vi "GUI_fast.vi"() -> ()   [LabVIEW 2013]
panel:
  out "indecator ref array":refnum<vi>[](array[refnum])
  in  "time to wait (TCP) 2":i32=10
  in  "plot":bool=TRUE
  out "ratio(h)":bool=TRUE
  out "fixsize":bool
  in  "shotnumber":i32
  out "error (h)":bool
  out "Device Name (h)":string="StagingOAP2Far"
  in  "Main Tap":T1(tab)
  in  "centroidx":dbl=453.118958
  in  "centroidy":dbl=178.22908
  out "XY Graph":cluster{u32, "centroidx":dbl}[](graph)=[{52, "centroidx"=458.85675}, {106, "centroidx"=457.702789}, {153, "centroidx"=451.882446}, {204, "centroidx"=452.284454}, {247, "centroidx"=452.532745}, {296, "centroidx"=451.082489}, {346, "centroidx"=459.559479}, {395, "centroidx"=451.41272}, {444, "centroidx"=452.080353}, {489, "centroidx"=451.756592}, {535, "centroidx"=455.360901}, {589, "centroidx"=451.727661}, {632, "centroidx"=457.428375}, {678, "centroidx"=458.708496}, {728, "centroidx"=456.774231}, {784, "centroidx"=457.488647}, {834, "centroidx"=451.875549}, {876, "centroidx"=457.952881}, {926, "centroidx"=459.627014}, {978, "centroidx"=456.600525}, {1024, "centroidx"=450.505829}, {1073, "centroidx"=452.936493}, {1123, "centroidx"=452.39035}, {1170, "centroidx"=452.66568}, {1219, "centroidx"=459.740845}, {1264, "centroidx"=426.268219}, {1316, "centroidx"=457.931732}, {1361, "centroidx"=457.714844}, {1411, "centroidx"=453.192993}, {1460, "centroidx"=456.957214}, {1508, "centroidx"=457.535095}, {1557, "centroidx"=459.828217}, {1602, "centroidx"=458.309296}, {1650, "centroidx"=457.216583}, {1697, "centroidx"=451.62738}, {1748, "centroidx"=457.94928}, {1794, "centroidx"=451.556854}, {1846, "centroidx"=454.358826}, {1890, "centroidx"=452.673492}, {1945, "centroidx"=457.183167}, {1992, "centroidx"=451.190216}, {2040, "centroidx"=457.415009}, {2091, "centroidx"=456.950653}, {2141, "centroidx"=458.052216}, {2186, "centroidx"=459.17218}, {2234, "centroidx"=458.392334}, {2287, "centroidx"=454.510315}, {2326, "centroidx"=458.260986}, {2378, "centroidx"=449.234619}, {2427, "centroidx"=452.183594}, {2473, "centroidx"=457.933685}, {2522, "centroidx"=458.143616}, {2568, "centroidx"=456.90979}, {2625, "centroidx"=453.549866}, {2675, "centroidx"=459.572571}, {2722, "centroidx"=456.521057}, {2768, "centroidx"=457.70401}, {2815, "centroidx"=457.971252}, {2862, "centroidx"=456.893097}, {2911, "centroidx"=452.007233}, {2960, "centroidx"=455.334778}, {3010, "centroidx"=457.899597}, {3057, "centroidx"=460.034424}, {3111, "centroidx"=456.625671}, {3149, "centroidx"=454.197052}, {3200, "centroidx"=453.378296}, {3250, "centroidx"=457.949677}, {3295, "centroidx"=453.204376}, {3349, "centroidx"=458.059357}, {3402, "centroidx"=451.967987}, {3448, "centroidx"=457.873352}, {3498, "centroidx"=449.439423}, {3537, "centroidx"=461.132538}, {3585, "centroidx"=458.034424}, {3641, "centroidx"=458.734589}, {3689, "centroidx"=450.626831}, {3737, "centroidx"=457.527283}, {3786, "centroidx"=458.842529}, {3826, "centroidx"=451.211609}, {3882, "centroidx"=459.017365}, {3932, "centroidx"=450.710937}, {3983, "centroidx"=453.03067}, {4027, "centroidx"=456.887268}, {4069, "centroidx"=457.095886}, {4121, "centroidx"=419.404022}, {4172, "centroidx"=459.245331}, {4219, "centroidx"=457.81781}, {4267, "centroidx"=457.769226}, {4319, "centroidx"=453.139252}, {4372, "centroidx"=457.15152}, {4409, "centroidx"=452.648102}, {4467, "centroidx"=459.761505}, {4507, "centroidx"=459.122864}, {4565, "centroidx"=451.026001}, {4606, "centroidx"=458.35379}, {4656, "centroidx"=457.762207}, {4702, "centroidx"=458.067657}, {4760, "centroidx"=456.013489}, {4797, "centroidx"=454.306244}, {4848, "centroidx"=450.459198}, {4893, "centroidx"=459.102936}, {4954, "centroidx"=450.82019}, {4994, "centroidx"=459.7099}, {5038, "centroidx"=459.12384}, {5093, "centroidx"=458.429321}, {5142, "centroidx"=459.938324}, {5192, "centroidx"=459.940643}, {5233, "centroidx"=458.946808}, {5283, "centroidx"=459.265167}, {5340, "centroidx"=457.806915}, {5380, "centroidx"=452.173462}, {5433, "centroidx"=452.593658}, {5474, "centroidx"=458.430847}, {5529, "centroidx"=460.566711}, {5577, "centroidx"=453.157745}, {5624, "centroidx"=457.170929}, {5677, "centroidx"=453.350372}, {5716, "centroidx"=457.141724}, {5776, "centroidx"=448.421906}, {5814, "centroidx"=460.143616}, {5872, "centroidx"=453.073975}, {5914, "centroidx"=458.349609}, {5963, "centroidx"=457.913513}, {6015, "centroidx"=453.412628}, {6058, "centroidx"=459.173279}, {6113, "centroidx"=458.18515}, {6158, "centroidx"=451.196808}, {6212, "centroidx"=459.467987}, {6250, "centroidx"=457.294434}, {6306, "centroidx"=456.740051}, {6347, "centroidx"=453.301453}, {6405, "centroidx"=457.164032}, {6454, "centroidx"=457.509949}, {6492, "centroidx"=456.408234}, {6542, "centroidx"=452.277863}, {6592, "centroidx"=452.098419}, {6643, "centroidx"=456.370667}, {6691, "centroidx"=459.323639}, {6739, "centroidx"=458.872498}, {6787, "centroidx"=458.552734}, {6841, "centroidx"=457.749664}, {6890, "centroidx"=453.448975}, {6932, "centroidx"=458.256073}, {6980, "centroidx"=459.461853}, {7025, "centroidx"=457.837555}, {7080, "centroidx"=453.918579}, {7122, "centroidx"=457.343475}, {7175, "centroidx"=456.631927}, {7225, "centroidx"=452.457184}, {7270, "centroidx"=459.418793}, {7321, "centroidx"=457.877014}, {7375, "centroidx"=457.096466}, {7420, "centroidx"=458.518066}, {7461, "centroidx"=458.402893}, {7512, "centroidx"=458.530121}, {7558, "centroidx"=456.802643}]
  in  "measure":bool
  out "local Port":u16=65420
  out "port or service name":u16=65419
  out "Remote Host":string="192.168.10.113"
  in  "timeout ms (slow resp)":i32=500
  in  "reset":bool
  out "image con closed":bool
  out "image \nconnection":bool
  out "image con closed 2":bool
  out "All Devices (h)":string[](array[string])=["B1_TelInput", "B6_SwitchYNear", "StagingDiodeMonitor", "StagingFocusBeam1", "StagingFocusBeam2", "StagingGuppy", "StagingM1Far", "StagingM1Near", "StagingM3Far", "StagingOAP1Far", "StagingOAP1Near", "StagingOAP2Far", "StagingOAP2Near", "TA6", "TS-ChromexCam", "TS-InputNearField", "TS-Mode1"]
  in  "time to wait (TCP)":i32=10
  out "error out":errorcluster
  out "connections (hidden)":variant[](array[variant])=[variant(refnum<k16> refnum), variant(refnum<k16> refnum)]
  in  "time to wait (main loop)":i32=10
  out "Data String":string="centroidy,178.229080\r\ncentroidx,453.118958\r\n"
  in  "Local Saving Path":path
  out "error message":string
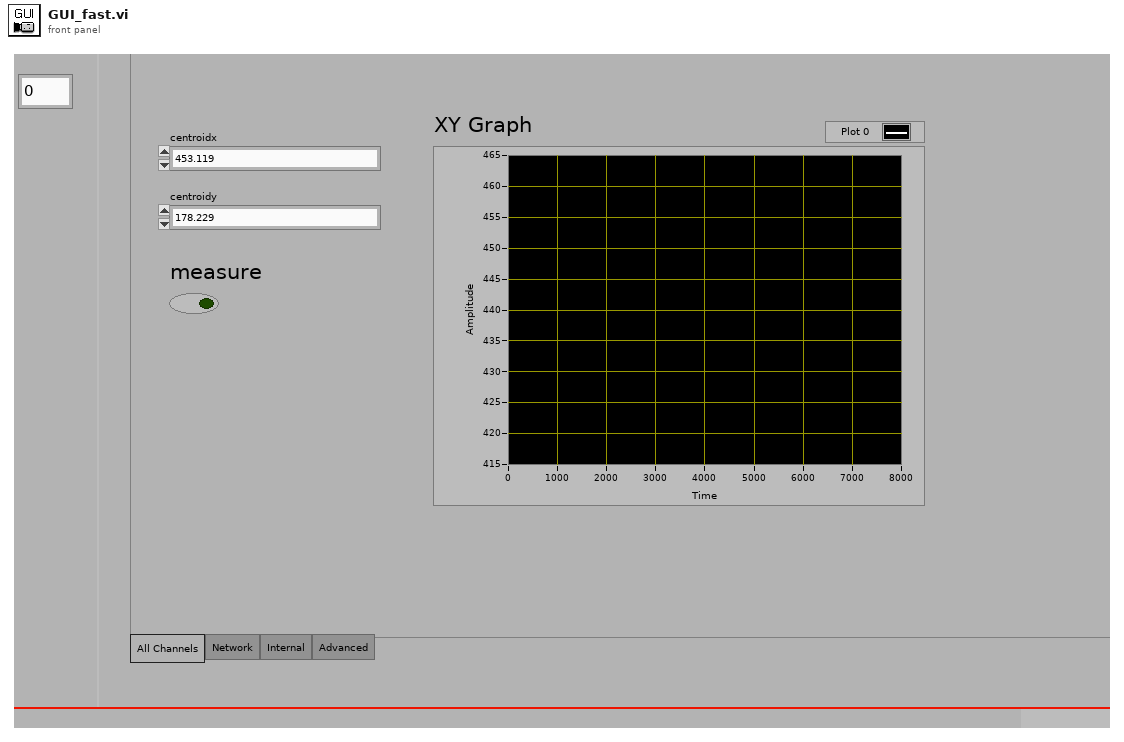
[diagram p1: front panel]
types:
  T1 = enum32{"All Channels", "Network", "Internal", "Advanced"}
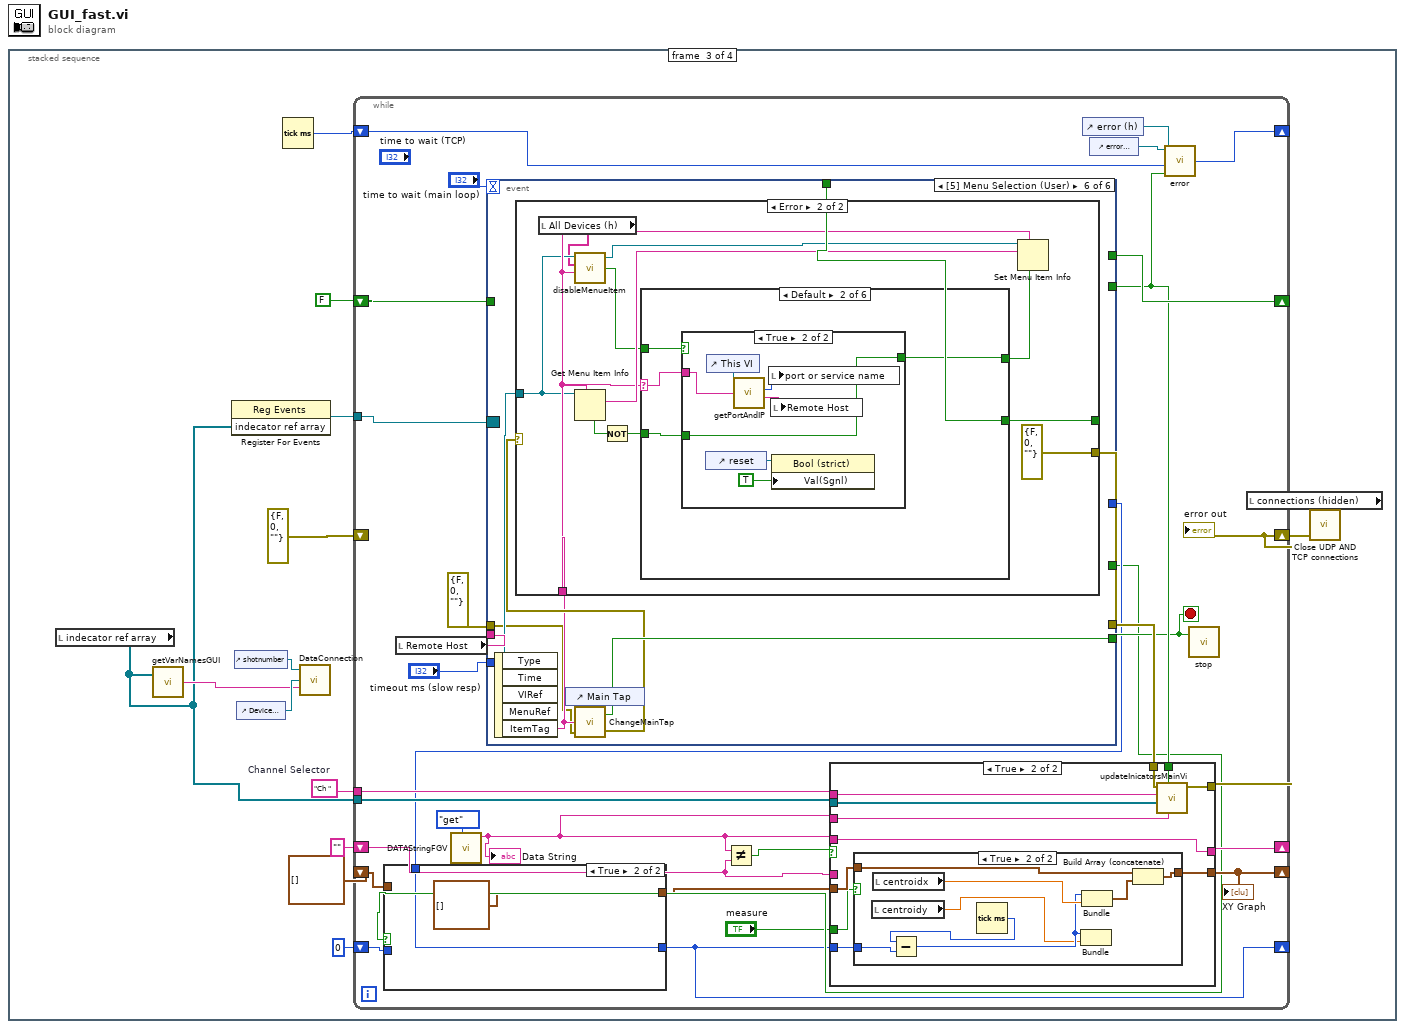
[diagram p0: block diagram]
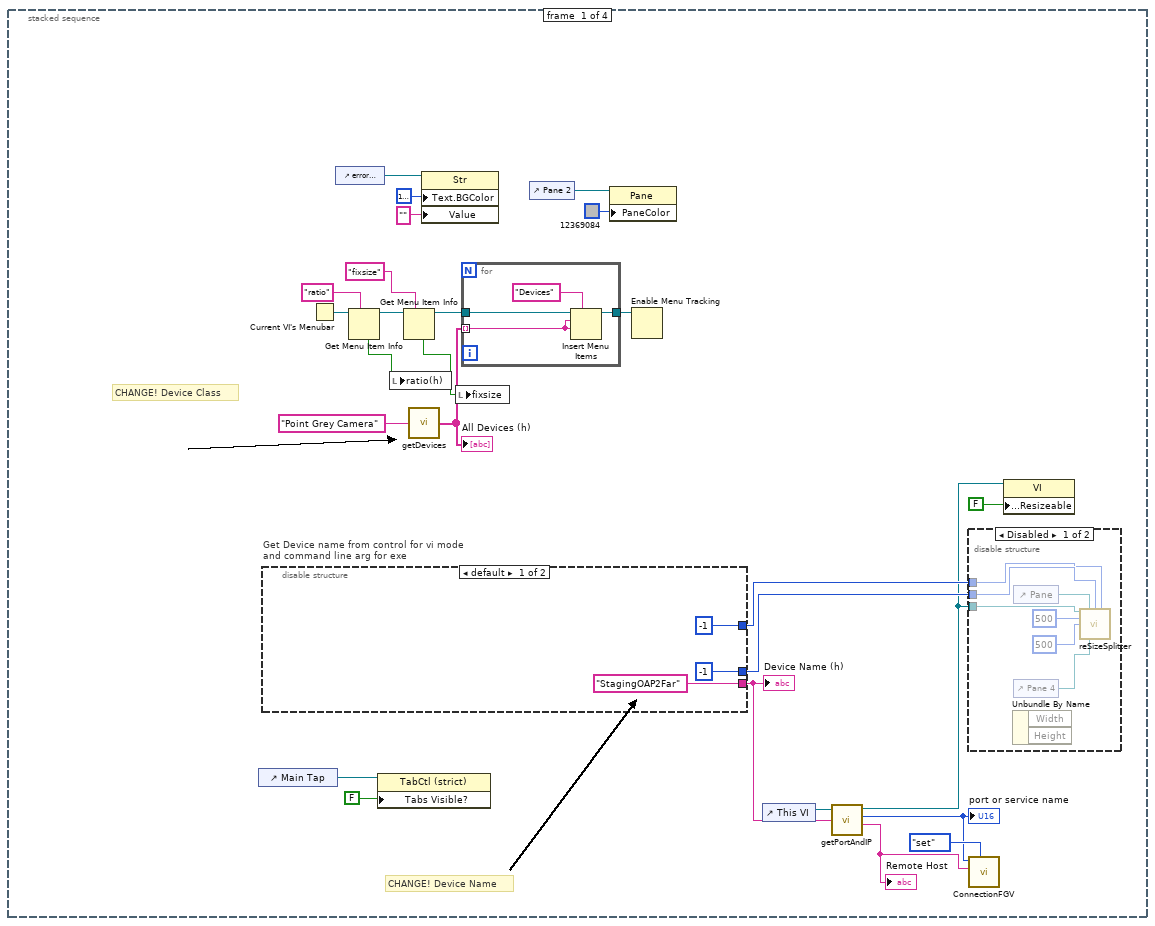
[diagram p2: hidden frame]
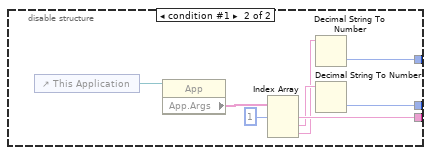
[diagram p4: hidden frame]
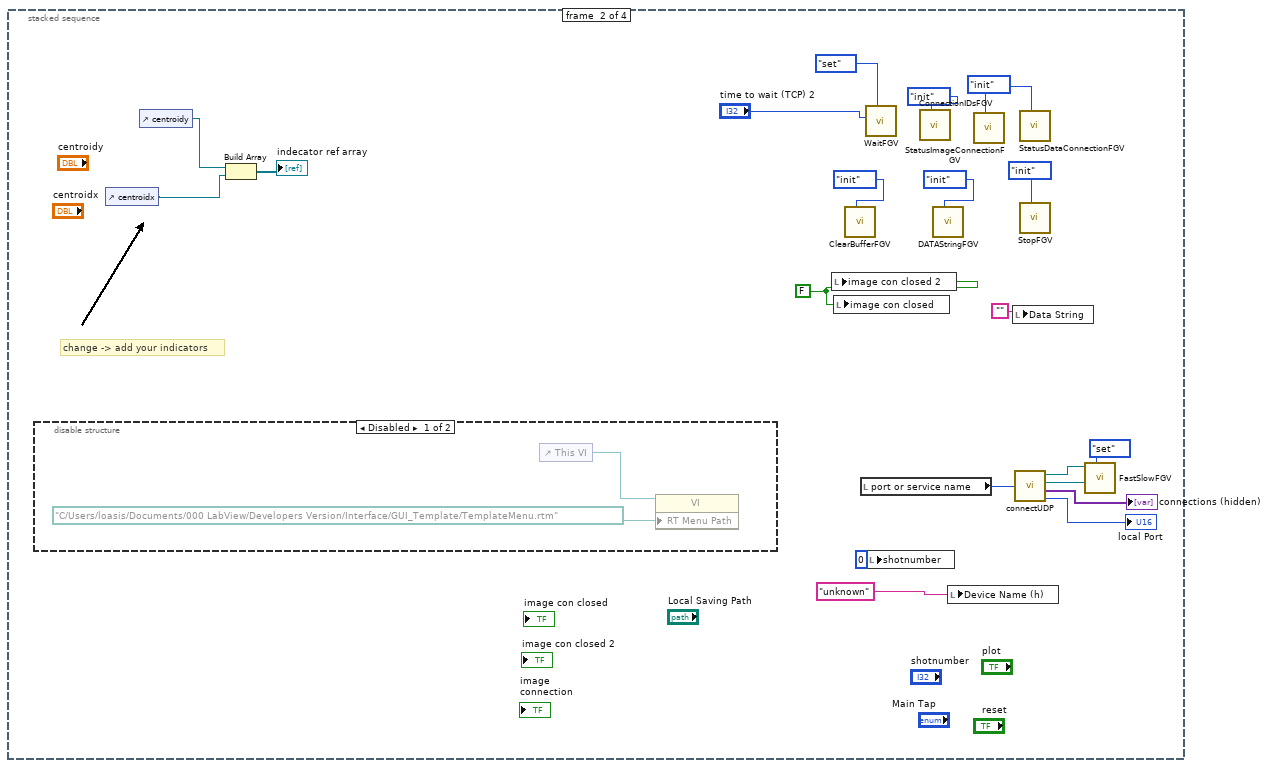
[diagram p5: hidden frame]
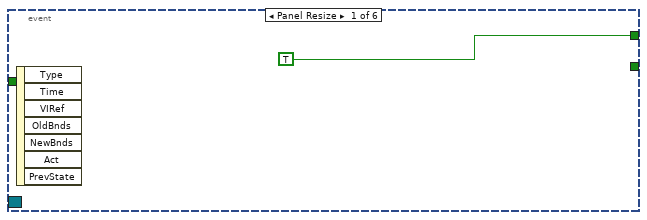
[diagram p10: hidden frame]
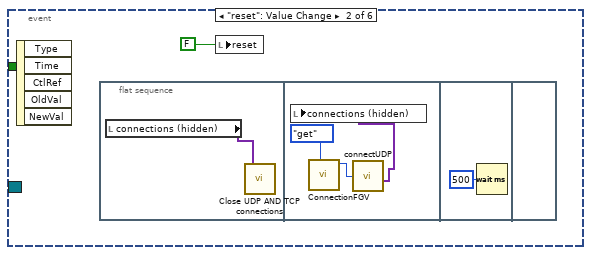
[diagram p11: hidden frame]
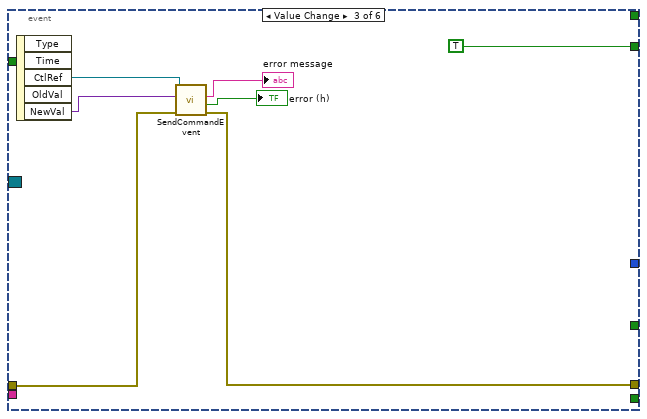
[diagram p12: hidden frame]
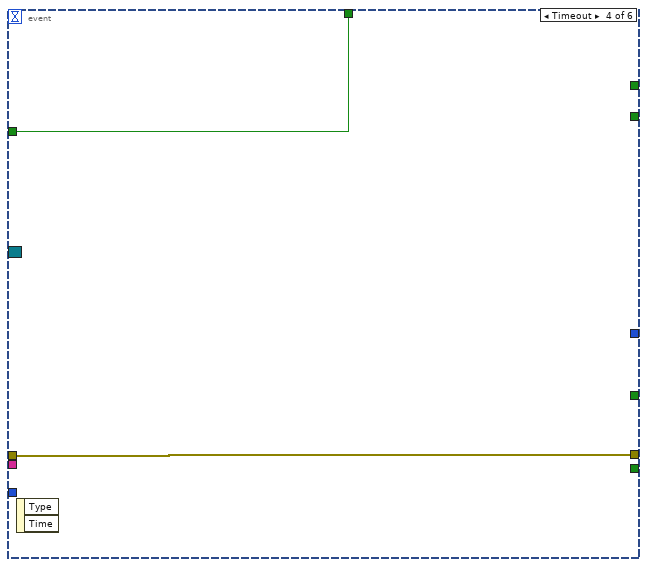
[diagram p13: hidden frame]
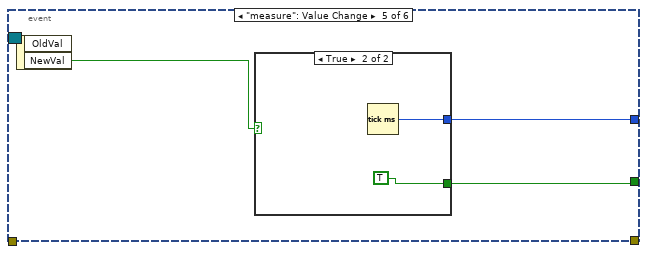
[diagram p14: hidden frame]
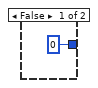
[diagram p15: hidden frame]
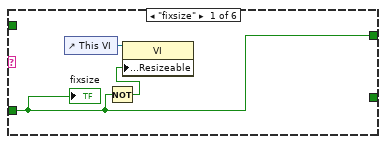
[diagram p17: hidden frame]
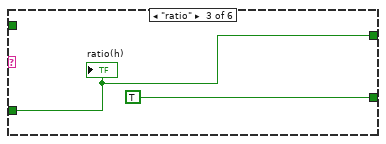
[diagram p19: hidden frame]
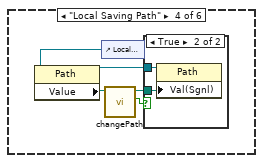
[diagram p20: hidden frame]
diagram:
  n1 = stacked-sequence {
    frame #0 {
      # "CHANGE! Device Name"
      # "CHANGE! Device Class"
      n2 = control-ref of="Main Tap"() -> (w26:refnum<vi>)
      n3 = disable-structure "Get Device name from control for vi mode\nand command line arg for exe" shown="default" {
        disable-tunnel: ["StagingOAP2Far" ("Device Name for vi mode") w45] -> w22
        disable-tunnel: [i16 -1 ("left") w42] -> w24
        disable-tunnel: [i16 -1 ("left") w41] -> w23
        frame condition #0 (active) {
        }
        frame condition #1 {
          n4 = control-ref of="This Application"() -> (w48:refnum<vi>)
          n5 = property class="App"(reference=w48) -> ("App.Args"=w47:string[])  [unwired: 1 in, 2 out]
          n6 = Index Array(array=w47, index #1=1 ("index")) -> (element #1=w45:string, element #2=w44:string, element #3=w43:string)  [unwired: 2 in]
          n7 = Decimal String To Number(string=w43) -> (number=w41:i32)  [unwired: 2 in, 1 out]
          n8 = Decimal String To Number(string=w44) -> (number=w42:i32)  [unwired: 2 in, 1 out]
        }
      }
      "Device Name (h)" <- w22
      n9 = Current VI's Menubar() -> (w7:refnum<k9>)
      n10 = control-ref of="error message"() -> (w14:refnum<vi>)
      n11 = Get Menu Item Info(7:"ratio" ("item tag"), 11:w7) -> (3:w5:refnum<k9>, 4:w6:bool)  [unwired: 1 in, 5 out]
      n12 = property class="TabCtl (strict)"(reference=w26, "Tabs Visible?"=FALSE) -> ()  [unwired: 1 in, 2 out]
      n13 = local write "ratio(h)"(w6) -> ()
      n14 = Get Menu Item Info(7:"fixsize" ("item tag"), 11:w5) -> (3:w2:refnum<k9>, 4:w3:bool)  [unwired: 1 in, 5 out]
      n15 = call "getDevices.vi"("Device Class"="Point Grey Camera") -> ("All Devices"=w10:string[])
      "All Devices (h)" <- w10
      n16 = property class="Str"(reference=w14, "Text.BGColor"=u32 16777238, "Value"="") -> ()  [unwired: 1 in, 2 out]
      n17 = local write "fixsize"(w3) -> ()
      n18 = for {
        tunnel: w2 -> [w30]
        tunnel: [w29] -> w1
        tunnel: w10 -> [w27] mode=indexing
        n19 = Insert Menu Items(5:"Devices" ("menu tag"), 7:w27, 8:w27, 9:w30) -> (3:w29:refnum<k9>)  [unwired: 2 in, 2 out]
      }
      n20 = control-ref of="Pane 2"() -> (w12:refnum<vi>)
      n21 = property class="Pane"(reference=w12, "PaneColor"=u32 12369084) -> ()  [unwired: 1 in, 2 out]
      n22 = Enable Menu Tracking(4:w1) -> ()  [unwired: 2 in, 2 out]
      n23 = control-ref of="This VI"() -> (w21:refnum<vi>)
      n24 = call "getPortAndIP.vi"("Device Name"=w22, "This Vi"=w21) -> ("Remote Host"=w17:string, "port or service name"=w16:u16, "reference out"=w19:refnum<vi>)  [unwired: 2 in, 2 out]
      "port or service name" <- w16
      "Remote Host" <- w17
      n25 = disable-structure shown="Disabled" {
        disable-tunnel: w24 -> [w36 _]
        disable-tunnel: w23 -> [w35 _]
        disable-tunnel: w19 -> [w33 _]
        frame Disabled {
          n26 = Unbundle By Name() -> ()  [unwired: 1 in, 2 out]
          n27 = control-ref of="Pane"() -> (w37:refnum<vi>)
          n28 = control-ref of="Pane 4"() -> (w34:refnum<vi>)
          n29 = call "reSizeSplitter.vi"("this vi"=w33, "pane"=w37, "left"=w36, "top"=w35, "Width"=u32 500, "Height"=u32 500, "pane2"=w34) -> ()  [unwired: 8 in, 1 out]
        }
        frame Enabled {
        }
      }
      n30 = call "ConnectionFGV.vi"("command"=enum16{"get", "set", "init"}."set", "Remote Host in"=w17, "port or service name in"=w16) -> ()  [unwired: 7 in, 2 out]
      n31 = property class="VI"(reference=w19, "Front Panel.Resizeable"=FALSE ("Front Panel Window:Resizable")) -> ()  [unwired: 1 in, 2 out]
    }
    frame #1 {
      w60 = enum16{"get", "set", "init"}."init" ("Command")
      w66 = FALSE ("new Device Data")
      # "change -> add your indicators"
      n32 = disable-structure shown="Disabled" {
        frame Disabled {
          n33 = control-ref of="This VI"() -> (w70:refnum<vi>)
          n34 = property class="VI"(reference=w70, "RT Menu Path"=path "C:/Users/loasis/Documents/000 LabView/Developers Version/Interface/GUI_Template/TemplateMenu.rtm" ("Run-Time Menu Path")) -> ()  [unwired: 1 in, 2 out]
        }
        frame Enabled {
        }
      }
      n35 = control-ref of="centroidx"() -> (w49:refnum<vi>)
      n36 = control-ref of="centroidy"() -> (w50:refnum<vi>)
      n37 = Build Array(w50, w49) -> (→"indecator ref array":refnum<vi>[])
      n38 = local write "image con closed 2"(w66) -> ()
      n39 = local write "image con closed"(w66) -> ()
      n40 = call "ClearBufferFGV.vi"("Command"=enum16{"set", "get", "init"}."init") -> ()  [unwired: 10 in, 1 out]
      n41 = local read "port or service name"() -> (w56:u16)
      n42 = call "WaitFGV.vi"("Command"=enum16{"get", "set", "init"}."set", "milliseconds to wait"="time to wait (TCP) 2") -> ()  [unwired: 9 in, 1 out]
      n43 = local write "shotnumber"(0 ("shotnumber")) -> ()
      n44 = call "ConnectionIDsFGV.vi"("Command"=enum16{"add", "get", "init"}."init") -> ()  [unwired: 10 in, 1 out]
      n45 = call "DATAStringFGV.vi"("Command"=enum16{"get", "set", "init"}."init") -> ()  [unwired: 9 in, 2 out]
      n46 = local write "Device Name (h)"("unknown" ("Device Name")) -> ()
      n47 = call "StatusImageConnectionFGV.vi"("Command"=w60) -> ()  [unwired: 10 in, 1 out]
      n48 = local write "Data String"("") -> ()
      n49 = call "connectUDP.vi"("port or service name NOT USED"=w56) -> ("fast ID (h)"=w55:refnum<k16>, "slow ID (h)"=w54:refnum<k16>, "connections (hidden)"=→"connections (hidden)":variant[], "local Port"=→"local Port":u16)
      n50 = call "StatusDataConnectionFGV.vi"("Command"=w60) -> ()  [unwired: 10 in, 1 out]
      n51 = call "StopFGV.vi"("Command"=enum16{"set", "get", "init"}."init") -> ()  [unwired: 9 in, 2 out]
      n52 = call "FastSlowFGV.vi"("Command"=enum16{"get", "set", "init"}."set", "slow ID"=w54, "fast ID"=w55) -> ()  [unwired: 7 in, 2 out]
    }
    frame #2 {
      w76 = "Ch "  # Channel Selector
      n53 = local read "indecator ref array"() -> (w74:refnum<vi>[])
      n54 = call "getVarNamesGUI.vi"("Array"=w74) -> ("String"=w75:string)  [unwired: 1 in]
      n55 = register-events(w74) -> (reference out=w77:refnum<event-registration>)  [unwired: 2 in, 1 out]
      n56 = control-ref of="shotnumber"() -> (w79:refnum<vi>)
      n57 = control-ref of="Device Name (h)"() -> (w78:refnum<vi>)
      n58 = Tick Count (ms)() -> (millisecond timer value=w80:u32)
      n59 = call "DataConnection.vi"("Subscriber list"=w75, "Device Name (h)"=w78, "shotnumber"=w79) -> ()
      n60 = while {
        shift-right: [w110] -> w83
        shift-left: errorcluster {"status"=FALSE, "code"=0, "source"=""} ("error out") -> [_]
        tunnel: w74 -> [w104]
        shift-right: [w108] -> _
        shift-left: FALSE -> [w109]
        shift-right: [w107] -> _
        shift-left: w80 -> [w106]
        tunnel: w77 -> [w101]
        tunnel: w76 -> [w100]
        shift-right: [w94] -> _
        shift-left: "" ("Data String out") -> [w93]
        shift-right: [w89] -> _
        shift-left: u32 0 ("millisecond timer value") -> [w88]
        shift-right: [w92] -> _
        shift-left: cluster{u32, "centroidx":dbl}[] [] -> [w86]
        stop <- w102 stop-if-true
        n61 = local read "Remote Host"() -> (w112:string)
        n62 = call "DATAStringFGV.vi"("Command"=enum16{"get", "set", "init"}."get") -> ("Data String out"=w95:string)  [unwired: 9 in, 1 out]
        "Data String" <- w95
        n63 = event shown="[5] Menu Selection (User)" {
          selector: w101 -> [_ _ _ _ _ _]
          dyn-events: _ -> [_ _ _ _ _ _]
          timeout: "time to wait (main loop)" -> [_ _ _ _ _ _]
          tunnel: [_ _ w153 w157 _ w165] -> w111
          tunnel: w112 -> [_ _ _ _ _ _]
          tunnel: "timeout ms (slow resp)" -> [_ _ _ _ _ _]
          tunnel: errorcluster {"status"=FALSE, "code"=0, "source"=""} ("error out") -> [_ _ w150 w157 _ w166]
          tunnel: [_ _ TRUE _ _ _] -> w105
          tunnel: [_ _ _ _ _ w171] -> w102
          tunnel: [_ _ _ w156 _ w168] -> _
          tunnel: w109 -> [_ _ _ w156 _ _]
          tunnel: [TRUE _ _ _ _ _] -> w108
          tunnel: [_ _ _ _ w160 _] -> w91
          tunnel: [_ _ _ _ w158 _] -> w90
          event Panel Resize {
            n64 = event-data() -> ()  [unwired: 1 in, 7 out]
          }
          event "reset": Value Change {
            n65 = event-data() -> ()  [unwired: 1 in, 5 out]
            n66 = flat-sequence {
              frame #0 {
                n67 = local read "connections (hidden)"() -> (w144:variant[])
                n68 = call "Close UDP AND TCP connections.vi"("appended array"=w144) -> ()  [unwired: 7 in]
              }
              frame #1 {
                n69 = call "ConnectionFGV.vi"("command"=enum16{"get", "set", "init"}."get") -> ("port or service name out"=w146:u16)  [unwired: 9 in, 1 out]
                n70 = call "connectUDP.vi"("port or service name NOT USED"=w146) -> ("connections (hidden)"=w145:variant[])  [unwired: 3 out]
                n71 = local write "connections (hidden)"(w145) -> ()
              }
              frame #2 {
                n72 = Wait (ms)(milliseconds to wait=u32 500) -> ()  [unwired: 1 out]
              }
              frame #3 {
              }
            }
            n73 = local write "reset"(FALSE ("reset")) -> ()
          }
          event Value Change {
            n74 = event-data() -> ("CtlRef"=w155:refnum<vi>, "NewVal"=w154:variant)  [unwired: 1 in, 3 out]
            n75 = call "SendCommandEvent.vi"("error out 2"=w150, "NewVal"=w154, "CtlRef"=w155) -> ("error out"=w153:errorcluster, "error (h)"=→"error (h)":bool, "error message"=→"error message":string)  [unwired: 5 in, 1 out]
          }
          event Timeout {
            n76 = event-data() -> ()  [unwired: 1 in, 2 out]
          }
          event "measure": Value Change {
            n77 = event-data() -> ("NewVal"=w159:bool)  [unwired: 1 in, 1 out]
            n78 = case shown="True" w159 {
              tunnel: [u32 0 ("millisecond timer value") w163] -> w160
              tunnel: [_ TRUE] -> w158
              frame False {
              }
              frame True {
                n79 = Tick Count (ms)() -> (millisecond timer value=w163:u32)
              }
            }
          }
          event Menu Selection (User) {
            n80 = event-data() -> ("MenuRef"=w167:refnum<k9>, "ItemTag"=w169:string)  [unwired: 1 in, 3 out]
            n81 = control-ref of="Main Tap"() -> (w164:refnum<vi>)
            n82 = call "ChangeMainTap.vi"("error in"=w166, "ItemTag"=w169, "reference"=w164) -> ("error out"=w170:errorcluster, "Boolean"=w171:bool)
            n83 = case shown="Error" w170 {
              selector: w170 -> [w172 _]
              tunnel: w167 -> [_ w178]
              tunnel: [_ w180] -> w168
              tunnel: w169 -> [_ w179]
              tunnel: [w172 errorcluster {"status"=FALSE, "code"=0, "source"=""} ("error IO")] -> w165
              frame No Error {
              }
              frame Error {
                n84 = local read "All Devices (h)"() -> (w173:string[])
                n85 = call "disableMenueItem.vi"("ItemTag"=w179, "All Devices (h)"=w173, "MenuRef"=w178) -> ("this is a Device(tag)"=w177:bool, "menu reference out"=w176:refnum<k9>)  [unwired: 1 in, 1 out]
                n86 = Get Menu Item Info(7:w179, 11:w178) -> (2:w182:string, 4:w183:bool)  [unwired: 1 in, 5 out]
                n87 = Not(x=w183) -> (.not. x?=w181:bool)
                n88 = case shown="Default" w179 {
                  selector: w179 -> [_ w189 _ _ _ _]
                  tunnel: w181 -> [w184 w187 w198 _ _ _]
                  tunnel: [_ _ TRUE _ _ _] -> w180
                  tunnel: w177 -> [_ w190 _ _ _ _]
                  tunnel: [w184 w188 w198 _ _ _] -> w175
                  frame "fixsize" {
                    n89 = control-ref of="This VI"() -> (w186:refnum<vi>)
                    n90 = Not(x=w184) -> (.not. x?=w185:bool)
                    n91 = property class="VI"(reference=w186, "Front Panel.Resizeable"=w185) -> ()  [unwired: 1 in, 2 out]
                    "fixsize" <- w184
                  }
                  frame Default {
                    n92 = case shown="True" w190 {
                      tunnel: w189 -> [_ w197]
                      tunnel: [_ w191] -> w188
                      tunnel: w187 -> [_ w191]
                      frame False {
                      }
                      frame True {
                        n93 = control-ref of="reset"() -> (w193:refnum<vi>)
                        n94 = control-ref of="This VI"() -> (w196:refnum<vi>)
                        n95 = call "getPortAndIP.vi"("Device Name"=w197, "This Vi"=w196) -> ("Remote Host"=w195:string, "port or service name"=w194:u16)  [unwired: 2 in, 3 out]
                        n96 = local write "port or service name"(w194) -> ()
                        n97 = local write "Remote Host"(w195) -> ()
                        n98 = property class="Bool (strict)"(reference=w193, "Val(Sgnl)"=TRUE ("Value (Signaling)")) -> ()  [unwired: 1 in, 2 out]
                      }
                    }
                  }
                  frame "ratio" {
                    "ratio(h)" <- w198
                  }
                  frame "Local Saving Path" {
                    n99 = control-ref of="Local Saving Path"() -> (w200:refnum<vi>)
                    n100 = property class="Path"(reference=w200) -> (reference out=w203:refnum<vi>, "Value"=w204:path)  [unwired: 1 in, 1 out]
                    n101 = call "changePath.vi"("Local Saving in (h)"=w204) -> ("change (h)"=w202:bool, "Local Saving out (h)"=w201:path)  [unwired: 9 in]
                    n102 = case shown="True" w202 {
                      tunnel: w203 -> [_ w206]
                      tunnel: w201 -> [_ w205]
                      frame False {
                      }
                      frame True {
                        n103 = property class="Path"(reference=w206, "Val(Sgnl)"=w205) -> ()  [unwired: 1 in, 2 out]
                      }
                    }
                  }
                  frame "reset" {
                    n104 = control-ref of="reset"() -> (w208:refnum<vi>)
                    n105 = property class="Bool (strict)"(reference=w208, "Val(Sgnl)"=TRUE ("Value (Signaling)")) -> ()  [unwired: 1 in, 2 out]
                  }
                  frame "clear" {
                    n106 = control-ref of="reset"() -> (w210:refnum<vi>)
                    n107 = property class="Bool (strict)"(reference=w210, "Val(Sgnl)"=TRUE ("Value (Signaling)")) -> ()  [unwired: 1 in, 2 out]
                  }
                }
                n108 = Set Menu Item Info(6:w175, 7:w179, 10:w182, 11:w176) -> ()  [unwired: 3 in, 2 out]
              }
            }
          }
        }
        n109 = case shown="True" w90 {
          tunnel: [w116 w118] -> w89
          tunnel: w91 -> [_ w118]
          tunnel: w88 -> [w116 _]
          tunnel: w86 -> [w115 _]
          tunnel: [w115 cluster{u32, "centroidx":dbl}[] []] -> w85
          frame False {
          }
          frame True {
          }
        }
        n110 = Not Equal?(x=w95, y=w93) -> (x != y?=w96:bool)
        n111 = case shown="True" w96 {
          tunnel: w111 -> [w120 w132]
          tunnel: [w120 w126] -> w110
          tunnel: w105 -> [_ w131]
          tunnel: w104 -> [_ w130]
          tunnel: w100 -> [_ w129]
          tunnel: w95 -> [_ w128]
          tunnel: w95 -> [_ w127]
          tunnel: [w121 w127] -> w94
          tunnel: w93 -> [w121 _]
          tunnel: w89 -> [_ w125]
          tunnel: [w119 w124] -> w92
          tunnel: w85 -> [w119 w123]
          tunnel: "measure" -> [_ w122]
          frame False {
          }
          frame True {
            n112 = case shown="True" w122 {
              tunnel: w125 -> [_ w134]
              tunnel: [w133 w137] -> w124
              tunnel: w123 -> [w133 w136]
              frame False {
              }
              frame True {
                n113 = local read "centroidy"() -> (w139:dbl)
                n114 = local read "centroidx"() -> (w141:dbl)
                n115 = Tick Count (ms)() -> (millisecond timer value=w135:u32)
                n116 = Subtract(x=w135, y=w134) -> (x-y=w140:u32)
                n117 = Bundle(w140, "centroidy"=w139) -> ()  [unwired: 1 in, 1 out]
                n118 = Bundle(w140, "centroidx"=w141) -> (w138:cluster{u32, "centroidx":dbl})  [unwired: 1 in]
                n119 = Build Array (concatenate)(w136, w138) -> (w137:cluster{u32, "centroidx":dbl}[])
              }
            }
            n120 = call "updateInicatorsMainVi.vi"("Data String out"=w128, "Boolean"=w131, "Array"=w130, "Channel Selector"=w129, "error in"=w132) -> ("error out"=w126:errorcluster)  [unwired: 4 in, 2 out]
          }
        }
        "error out" <- w110
        "XY Graph" <- w92
        n121 = control-ref of="error (h)"() -> (w97:refnum<vi>)
        n122 = control-ref of="error message"() -> (w98:refnum<vi>)
        n123 = call "error.vi"("Boolean"=w105, "millisecond timer value"=w106, "reference"=w97, "error message"=w98) -> ("millisecond timer value 2"=w107:u32)
        n124 = call "stop.vi"("Boolean"=w102) -> ()
      }
      n125 = local read "connections (hidden)"() -> (w82:variant[])
      n126 = call "Close UDP AND TCP connections.vi"("error in"=w83, "appended array"=w82) -> ()  [unwired: 6 in]
    }
    frame #3 {
      n127 = control-ref of="Main  Control"() -> (w212:refnum<vi>)
      n128 = property class="TabCtl (strict)"(reference=w212, "Tabs Visible?"=TRUE) -> ()  [unwired: 1 in, 2 out]
      n129 = property class="TabCtl (strict)"(reference=w212, "Tab Location"=enum32{"Top", "Bottom", "Left", "Right"}."Bottom") -> ()  [unwired: 1 in, 2 out]
      n130 = flat-sequence {
        frame #0 {
          n131 = Wait (ms)(milliseconds to wait=u32 0) -> ()  [unwired: 1 out]
        }
        frame #1 {
        }
        frame #2 {
          n132 = control-ref of="This VI"() -> (w217:refnum<vi>)
          n133 = case shown="True" FALSE {
            tunnel: w217 -> [w218 w221]
            tunnel: [w218 w219] -> w216
            frame False {
            }
            frame True {
              n134 = property class="VI" props=["Front Panel.Open"](reference=w221) -> (reference out=w220:refnum<vi>)  [unwired: 1 in, 2 out]
              n135 = invoke class="VI" method="FP.Close"(reference=w220) -> (reference out=w219:refnum<vi>)  [unwired: 2 in, 2 out]
            }
          }
          n136 = Close Reference(reference=w216) -> ()  [unwired: 1 in, 1 out]
        }
      }
    }
  }
